vi "5.7-Reliable UDP Server Template.vi"() -> ()   [LabVIEW 2010]
doc: "UDP Mutlicast Addressing Scheme:\n\n3.7 - Multicast Address: 133.7.3.7\n3.1-4.7.1 Port: 31471\n3.2-4.7.2 Port: 32472\n3.3-4.7.3 Port: 33473\n3.4-4.7.4 Port: 34474\n\n5.7 - Multicast Address: 133.7.5.7\n5.1-4.7.1 Port: 51471\n5.2-4.7.2 Port: 52472\n5.3-4.7.3 Port: 53473\n5.4-4.7.4 Port: 54474\n\n5.1-6.7.1 Port: 51671\n5.2-6.7.2 Port: 52672\n5.3-6.7.3 Port: 53673\n5.4-6.7.4 Port: 54674\n\n7.7 - Multicast Address: 133.7.7.7\n7.1-6.7.1 Port: 61671\n7.2-6.7.2 Port: 62672\n7.3-6.7.3 Port: 63673\n7.4-6.7.4 Port: 64674"
uses:
  4-High Neurons/4.0-Timing Badass.ctl
  <vilib>/Utility/tcp.llb/UDP Multicast Write-Only Open.vi
  5.0-Global.vi
panel:
  out "Super Heart Beat 2":T1
  out "Error":errorcluster
  in  "stop":bool
  out "Processed":string
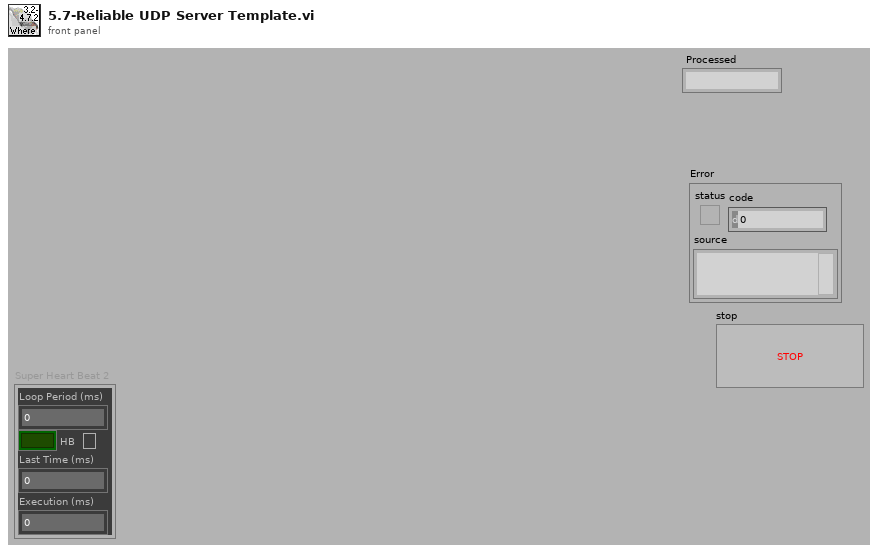
[diagram p1: front panel]
types:
  T1 = typedef "4.0-Timing Badass.ctl" = cluster{"Loop Period (ms)":u32, "HB":bool, "Last Time (ms)":u32, "Execution (ms)":u32}
  T2 = typedef "4.1-Act Control Typedef.ctl" = cluster{"4.1.0 Data":variant, "Type of Data":T3, "E-Stop":bool, "Restart":bool, "New IP":bool, "Begin":bool, "Time":i32, "Shutdown":bool}
  T3 = typedef "4.1.0-Datatype Typedef.ctl" = enum16{"4.1.0-Empty Data", "4.1.1-Joystick Data", "4.1.2-Behavioral Data"}
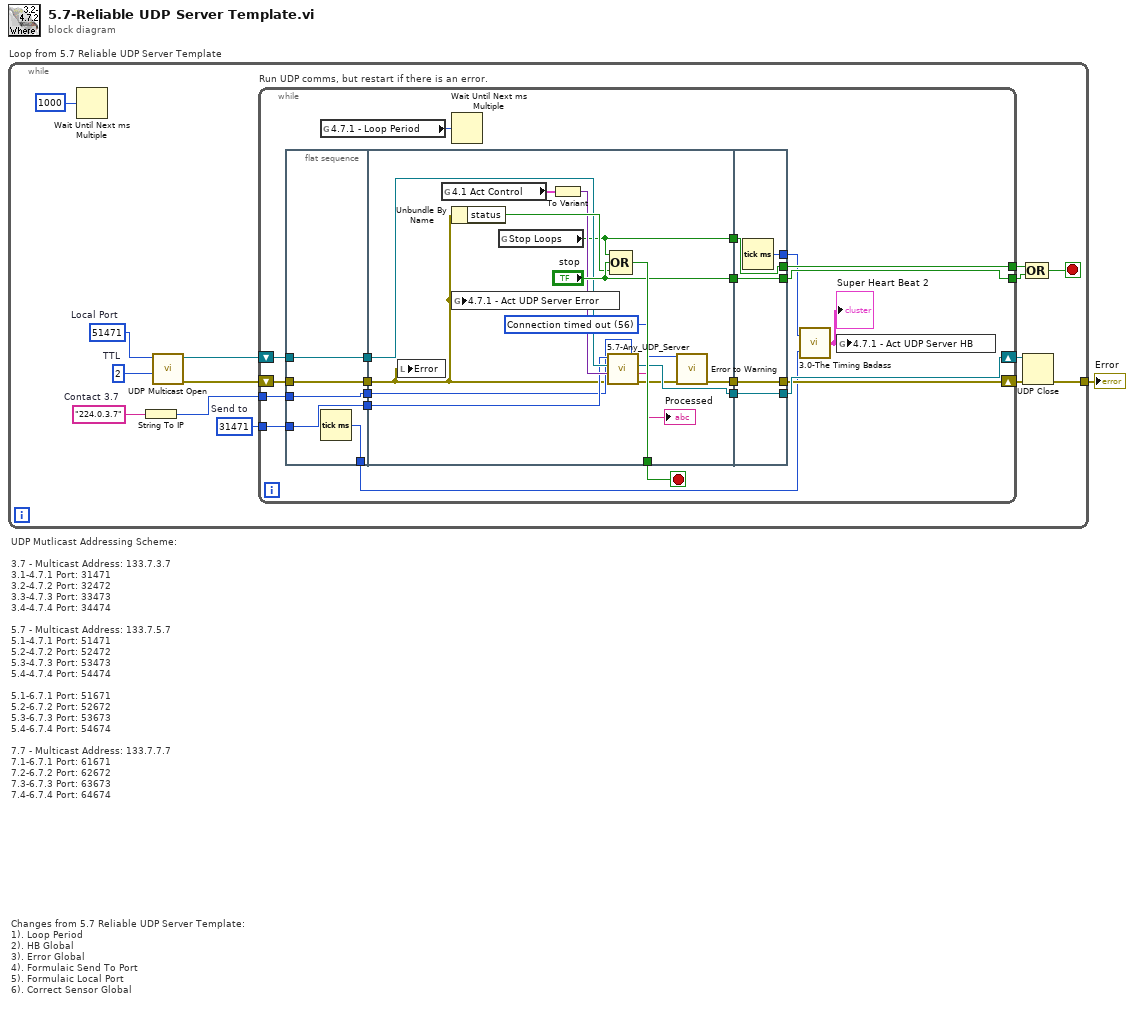
[diagram p0: block diagram]
diagram:
  # "Changes from 5.7 Reliable UDP Server Template:\n1). Loop Period\n2). HB Global\n3). Error Global\n4). Formulaic Send To Port\n5). Formulaic Local Port\n6). Correct Sensor Global"
  # "UDP Mutlicast Addressing Scheme:\n\n3.7 - Multicast Address: 133.7.3.7\n3.1-4.7.1 Port: 31471\n3.2-4.7.2 Port: 32472\n3.3-4.7.3 Port: 33473\n3.4-4.7.4 Port: 34474\n\n5.7 - Multicast Address: 133.7.5.7\n5.1-4.7.1 Port: 51471\n5.2-4.7.2 Port: 52472\n5.3-4.7.3 Port: 53473\n5.4-4.7.4 Port: 54474\n\n5.1-6.7.1 Port: 51671\n5.2-6.7.2 Port: 52672\n5.3-6.7.3 Port: 53673\n5.4-6.7.4 Port: 54674\n\n7.7 - Multicast Address: 133.7.7.7\n7.1-6.7.1 Port: 61671\n7.2-6.7.2 Port: 62672\n7.3-6.7.3 Port: 63673\n7.4-6.7.4 Port: 64674"
  n1 = while "Loop from 5.7 Reliable UDP Server Template" {
    tunnel: [w10] -> w1
    stop <- w13 stop-if-true
    w2 = "224.0.3.7"  # Contact 3.7
    w4 = u16 31471  # Send to
    w7 = u16 2  # TTL
    w8 = u16 51471  # Local Port
    n2 = Wait Until Next ms Multiple(millisecond multiple=u32 1000) -> ()  [unwired: 1 out]
    n3 = String To IP(1:w2) -> (0:w3:u32)
    n4 = call-poly <vilib>:"UDP Multicast Open.vi"("time-to-live (1)"=w7, "port"=w8) -> ("error out"=w5:errorcluster, "connection ID"=w6:refnum<k16>)  [unwired: 8 in]
    n5 = while "Run UDP comms, but restart if there is an error." {
      tunnel: [w29] -> w15
      tunnel: [w35] -> w14
      shift-right: [w33] -> w12
      shift-left: w6 -> [w34]
      shift-right: [w30] -> w11
      shift-left: w5 -> [w27]
      tunnel: w4 -> [w32]
      tunnel: w3 -> [w31]
      stop <- w36 stop-if-true
      n6 = flat-sequence {
        tunnel: w27 -> [w38]
        tunnel: w31 -> [w39]
        tunnel: w32 -> [w40]
        tunnel: w34 -> [w41]
        tunnel: [w41] -> w22
        tunnel: [w40] -> w21
        tunnel: [w39] -> w20
        tunnel: [w38] -> w19
        tunnel: [w37] -> w18
        tunnel: [w56] -> w36
        tunnel: ["stop"] -> w26
        tunnel: [w49] -> w25
        tunnel: [w44] -> w24
        tunnel: [w43] -> w23
        tunnel: w22 -> [w50]
        tunnel: w21 -> [w48]
        tunnel: w20 -> [w47]
        tunnel: w19 -> [w42]
        tunnel: [w58] -> w29
        tunnel: [w59] -> w30
        tunnel: [w60] -> w33
        tunnel: [w61] -> w35
        tunnel: w26 -> [w61]
        tunnel: w25 -> [w60]
        tunnel: w24 -> [w59]
        tunnel: w23 -> [w58]
        tunnel: [w57] -> w17
        frame #0 {
          n7 = Tick Count (ms)() -> (millisecond timer value=w37:u32)
        }
        frame #1 {
          w45 = 56 items=["No Error", "Argument Error", "Memory Full", "Out of Zone", "End of File", "File Already Open", "Generic File IO Error", "File Not Found", "File Permission Error", "Disk Full", "Duplicate Path", "Too Many Files Open", "Not Enabled", "Resource File Not Found", "Cannot Add Resource", "Resource Not Found", "Image Not Found", "Image Memory Error", "Pen Does Not Exist", "Config Bad Type", "Config Token Not Found", "Config Parse Error", "Config Memory Error", "Bad External Code Format", "Bad External Code Offset", "External Code Not Present", "Null Window", "Destroy Window Mixup", "Null Menu", "Print Aborted", "Bad Print Record", "Print Driver Error", "Windows Error During Print", "Memory Error During Print", "Print Dialog Error", "Generic Print Error", "Invalid Device Refnum", "Device Not Found", "Device Parameter Error", "Device Unit Error", "Can't Open Device", "Device Call Aborted", "Generic Error", "Cancelled By User", "Object ID Too Low", "Object ID Too High", "Object Not In Heap", "Unknown Heap", "Bad DefProc ID", "DefProc Not In Table", "Message Out Of Range", "Null Method", "Unknown Message", "Manager Call Not Supported", "Bad address", "Connection In progress", "Connection timed out", "Connection is already in progress", "Network attribute not supported", "Network error", "Address in use", "System out of memory", "Connection aborted", "Connection refused", "Connection is not connected", "Connection is already connected", "Connection closed", "Initialize error (interapplication manager)", "Bad occurrence", "Wait on unbound occurrence handler", "Occurrence queue overflow", "Bad path", "Semaphore not signaled", "Unrecognized type (interapplication manager)"] ("1st Error to Convert")
          n8 = local write "Error"(w42) -> ()
          n9 = global read "5.0-Global.vi" "4.1 Act Control"() -> (w52:T2)
          n10 = Unbundle By Name(w42) -> ("status"=w54:bool)
          n11 = global write "5.0-Global.vi" "4.7.1 - Act UDP Server Error"(w42) -> ()
          n12 = global read "5.0-Global.vi" "Stop Loops"() -> (w43:bool)
          n13 = To Variant(anything=w52) -> (Variant=w53:variant)
          n14 = call "5.7-Any_UDP_Server.vi"("Multicast Address"=w47, "error In"=w42, "Data in"=w53, "Connection ID"=w50, "Send To Port"=w48) -> ("warning out"=w46:errorcluster, "Processed"=→"Processed":string, "Connection ID out"=w49:refnum<k16>)
          n15 = Compound Arithmetic op=OR(w43, "stop", w54) -> (w56:bool)
          n16 = call <vilib>:"Error to Warning.vi"("1st Error to Convert"=w45, "error in"=w46) -> ("warning out"=w44:errorcluster)  [unwired: 13 in]
        }
        frame #2 {
          n17 = Tick Count (ms)() -> (millisecond timer value=w57:u32)
        }
      }
      n18 = global read "5.0-Global.vi" "4.7.1 - Loop Period"() -> (w28:u32)
      n19 = Wait Until Next ms Multiple(millisecond multiple=w28) -> ()  [unwired: 1 out]
      n20 = call "3.0-The Timing Badass.vi"("Start"=w18, "End"=w17) -> ("Super Heart Beat"=w16:T1)
      "Super Heart Beat 2" <- w16
      n21 = global write "5.0-Global.vi" "4.7.1 - Act UDP Server HB"(w16) -> ()
    }
    n22 = UDP Close(connection ID=w12, 8:w11) -> (error out=w10:errorcluster)  [unwired: 1 out]
    n23 = Compound Arithmetic op=OR(w15, w14) -> (w13:bool)
  }
  "Error" <- w1
